vi "vPage_9234x1_CHx4_demo.vi"() -> ()   [LabVIEW 2022 SP3]
uses:
  <vilib>/Utility/sysdir.llb/System Directory Type.ctl
  <vilib>/express/express analysis/Spectral/Block/exnSpectralBlock spectral measurements peak poly.vi
  <vilib>/express/express analysis/Spectral/Block/exnSpectralBlock spectral measurements peak DDT.vi
  <vilib>/express/express analysis/Spectral/XNode/ExpressSpectralMeasurementsBlockNode.xnode
panel:
  out "SPC ALARM":bool
  in  "MTIG":bool
  out "C1":i32
  in  "Show_FFT":bool
  in  "Show":bool
  in  "¸ê®Æ§¨\nµù°O>":string
  in  "Filter(Hz)\nLow-Cut":dbl=10.0
  out "DAQ Stoped":bool
  in  "Sample \nto Read":i32=25600
  in  "Sample\nRate":dbl=25600.0
  in  "Enable Saving":bool
  in  "Stop":bool
  out "C1-Save":bool
  out "C1-Trigger":bool
  out "C1-All":dynamicdata(graph)
  out "C1-0":dynamicdata(graph)
  out "C1-1":dynamicdata(graph)
  out "C1-2":dynamicdata(graph)
  out "C1-3":dynamicdata(graph)
  out "RMS":T1(graph)
  out "P2P":T1(graph) caption="Peak2Peak"
  out "疊層訊號":dbl[][](graph)
  # "使用前請先確認 \nDAQ 擷取卡設定"
  # "本頁畫面顯示為 觸發後訊號"
  # "FFT Filter by useing High-pass with Lower Cut-Off (Hz)"
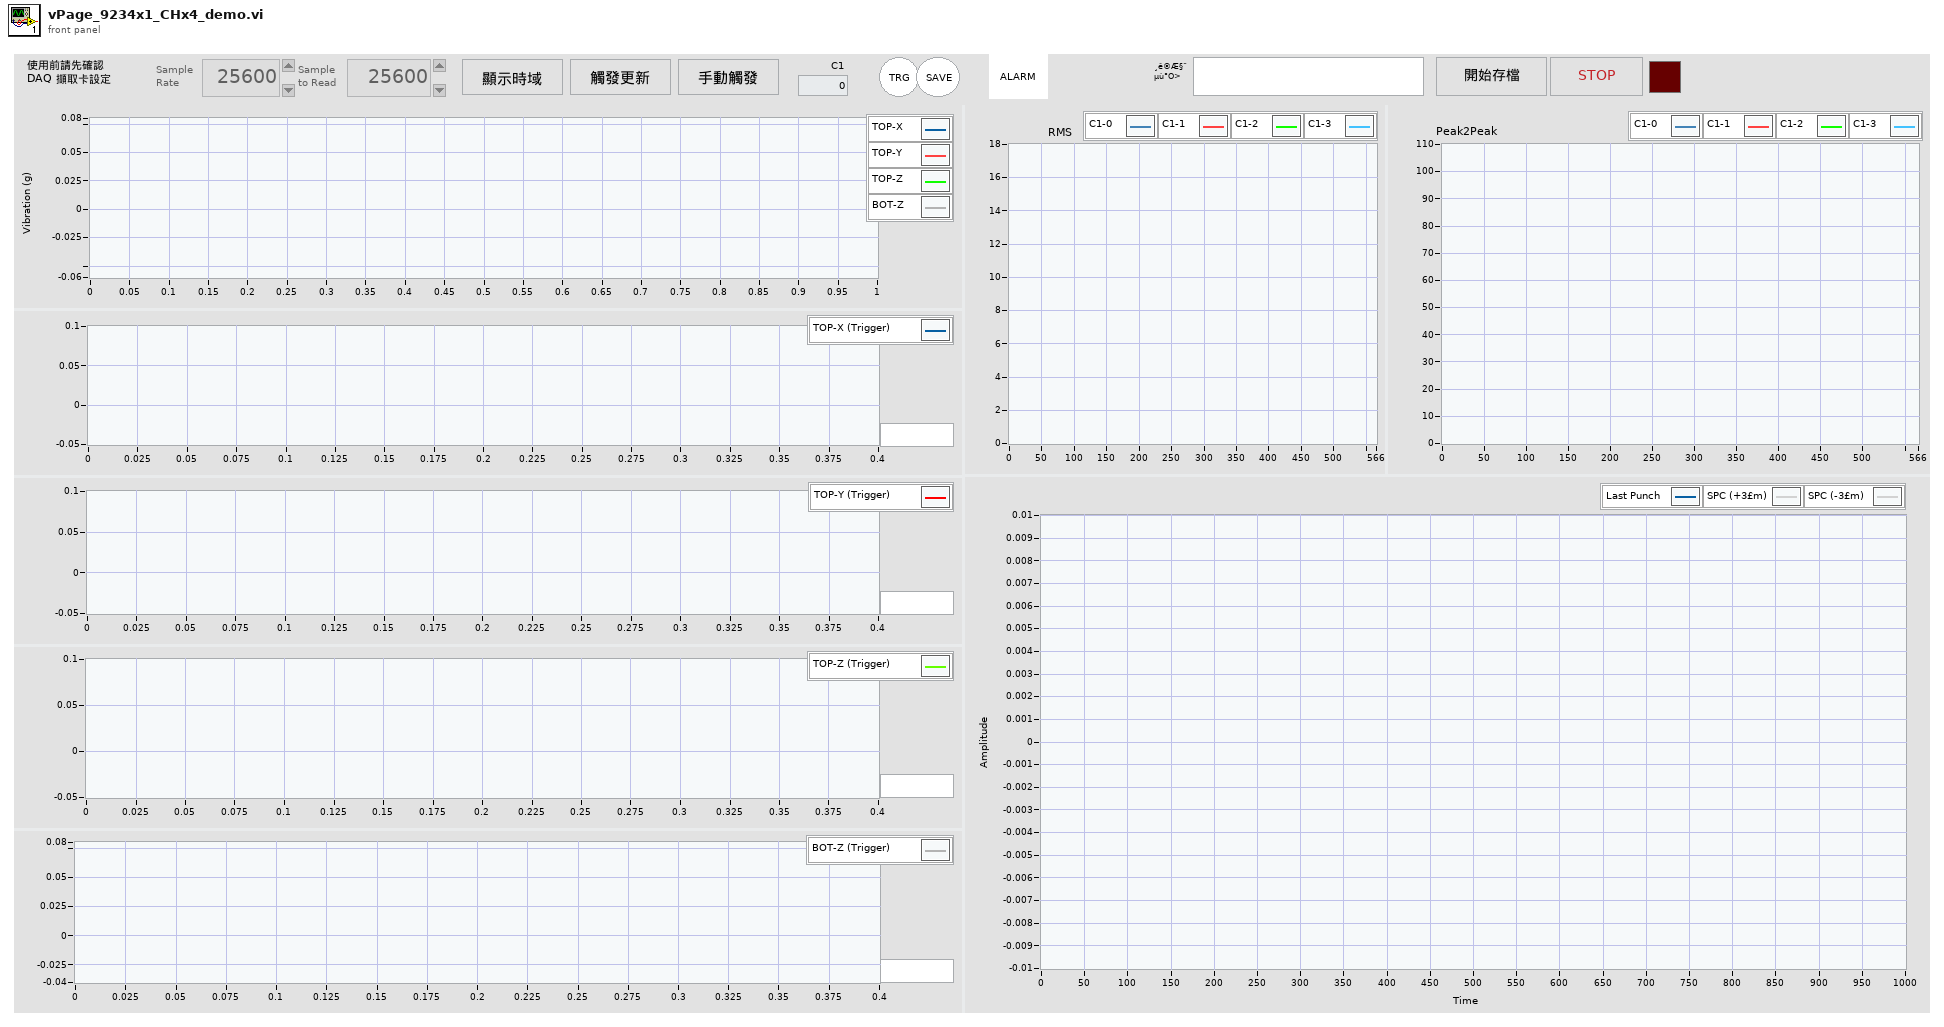
[diagram p1: front panel]
types:
  T1 = cluster{"Array[0]":dbl, "Array[1]":dbl, "Array[2]":dbl, "Array[3]":dbl}
  T2 = enum8{"Enabled", "Disabled", "Disabled and Grayed Out"}
  T3 = typedef "System Directory Type.ctl" = i32
  T4 = cluster{"task out":refnum<k21>, "data":dynamicdata}
  T5 = cluster{"averaging mode":u16, "weighting mode":u16, "number of averages":u32}
  T6 = cluster{"dB On (F)":bool, "unwrap phase (F)":bool, "convert to degree (F)":bool}
  T7 = cluster{"Array[0]":dbl, "Array[1]":dbl, "Array[2]":dbl, "Array[3]":dbl}[]
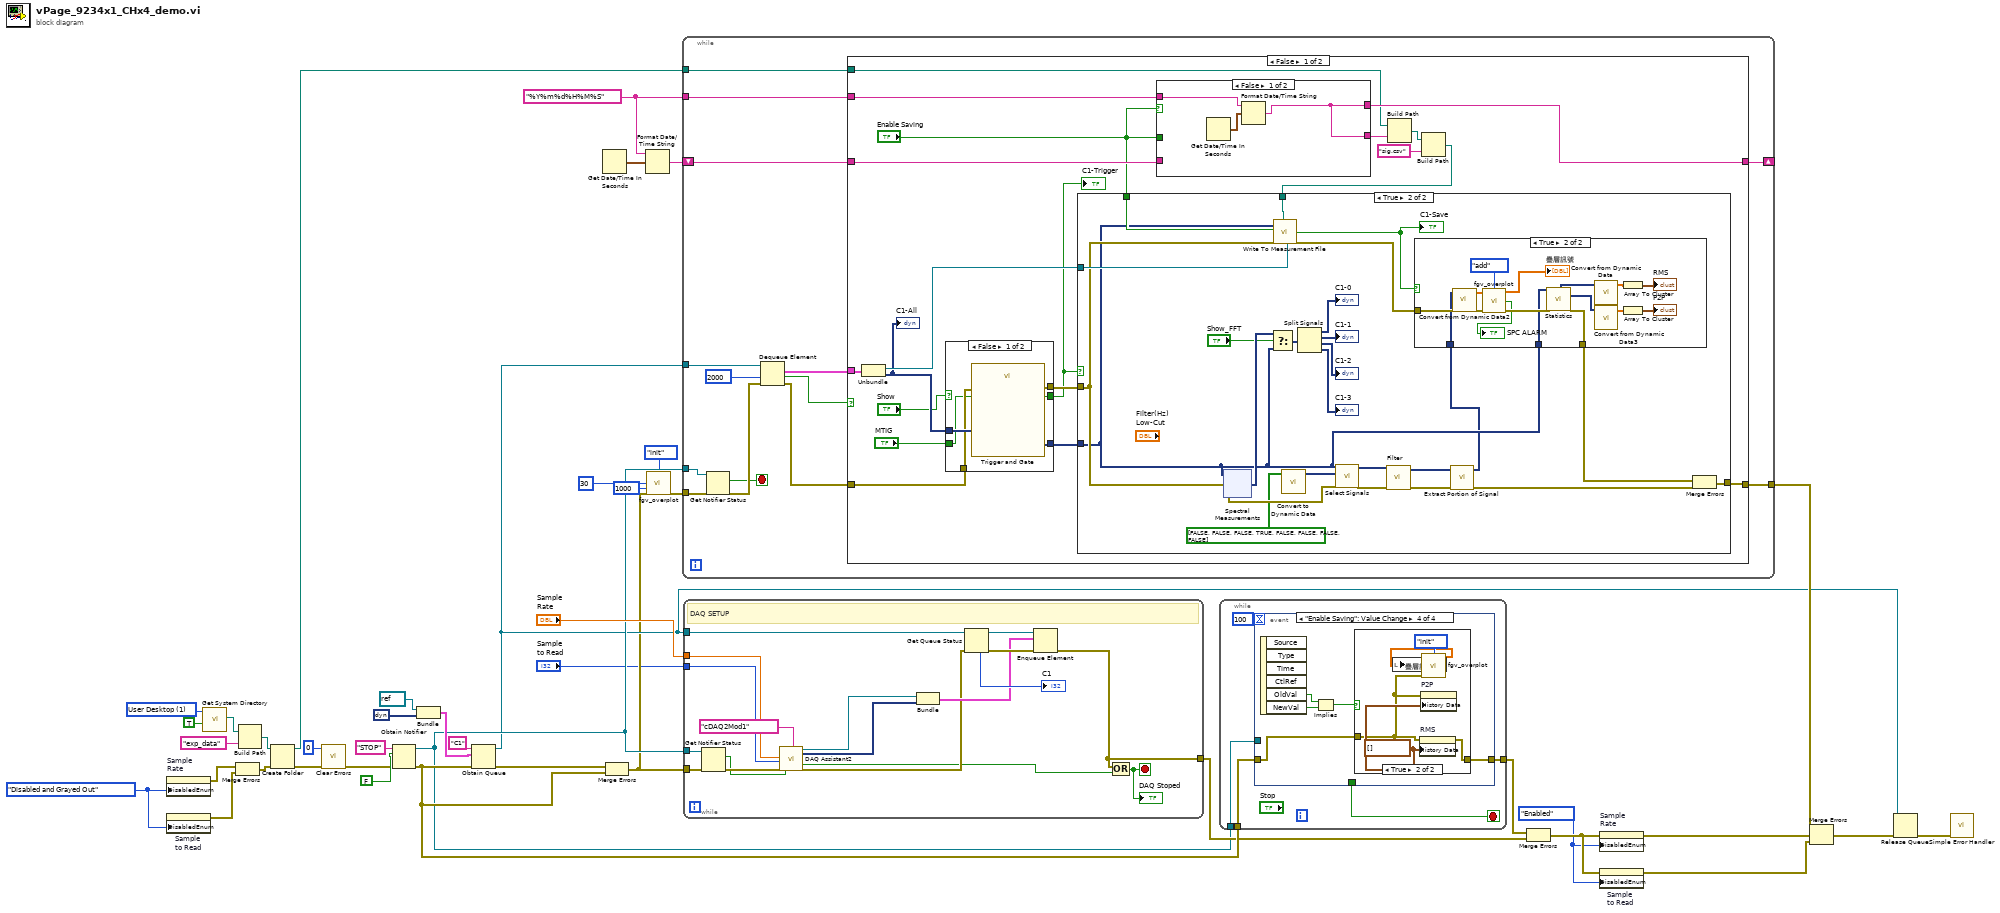
[diagram p0: block diagram]
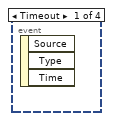
[diagram p2: hidden frame]
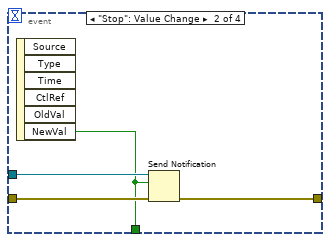
[diagram p3: hidden frame]
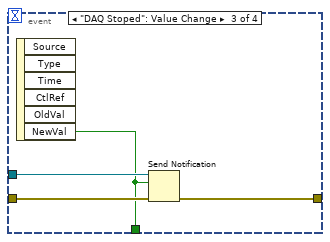
[diagram p4: hidden frame]
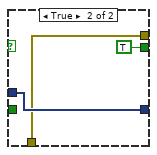
[diagram p8: hidden frame]
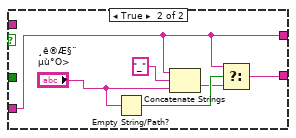
[diagram p9: hidden frame]
diagram:
  w13 = T2."Enabled" ("Disabled")
  w18 = T2."Disabled and Grayed Out" ("Disabled")
  w19 = "%Y%m%d%H%M%S" ("time format string (%c)")
  w29 = T3 1 items=["User Home"=0, "User Desktop"=1, "User Documents"=2, "User Application Data"=3, "User Preferences"=4, "User Temporary"=5, "Public Documents"=6, "Public Application Data"=7, "Public Preferences"=8, "Public Cache"=13, "System Core Libraries"=9, "System Installed Libraries"=10, "Application Files"=11, "Boot Volume Root"=12] ("system directory type")
  n1 = property on="Sample\nRate" class="DigNum (strict)"("DisabledEnum"=w18) -> (error out=w17:errorcluster)  [unwired: 2 in, 1 out]
  n2 = property on="Sample \nto Read" class="DigNum (strict)"("DisabledEnum"=w18) -> (error out=w15:errorcluster)  [unwired: 2 in, 1 out]
  n3 = call <vilib>:"Get System Directory.vi"("create directory if not found? (F)"=TRUE, "system directory type"=w29) -> ("system directory"=w31:path)  [unwired: 9 in]
  n4 = Merge Errors(w17, w15) -> (w16:errorcluster)
  n5 = Build Path(base path=w31, name or relative path="exp_data") -> (appended path=w25:path)
  n6 = Create Folder(path (use dialog)=w25, error in=w16) -> (created path=w24:path, error out=w27:errorcluster)  [unwired: 1 in, 1 out]
  n7 = call <vilib>:"Clear Errors.vi"("error in (no error)"=w27, "specific error code to clear (0: all)"=0) -> ("error out"=w26:errorcluster)  [unwired: 4 in, 1 out]
  n8 = Obtain Notifier(name (unnamed)="STOP", notification data type=FALSE, error in (no error)=w26) -> (notifier out=w20:refnum<notifier>, error out=w23:errorcluster)  [unwired: 1 in, 1 out]
  n9 = Bundle("task out"=refnum<k21> refnum, "data"=dynamicdata []) -> (w35:T4)  [unwired: 1 in]
  n10 = Obtain Queue(name (unnamed)="C1", element data type=w35, error in (no error)=w23) -> (queue out=w7:refnum<queue>, error out=w42:errorcluster)  [unwired: 2 in, 1 out]
  n11 = Get Date/Time In Seconds() -> (seconds since 1Jan1904=w34:timestamp)
  n12 = Merge Errors(w42, w23) -> (w5:errorcluster)
  n13 = Format Date/Time String(time format string (%c)=w19, seconds (now)=w34) -> (date/time string=w33:string)  [unwired: 1 in]
  n14 = call "fgv_overplot.vi"("function (default: show)"=enum16{"init", "add"}."init", "num for avg"=u32 30, "total samples"=u32 1000, "error in"=w5) -> ("error out"=w4:errorcluster)  [unwired: 9 in, 2 out]
  n15 = while {
    tunnel: w4 -> [w56]
    tunnel: w20 -> [w54]
    tunnel: w7 -> [w53]
    shift-right: [w43] -> _
    shift-left: w33 -> [w47]
    tunnel: w24 -> [w48]
    tunnel: [w44] -> w8
    tunnel: w19 -> [w46]
    stop <- w51 stop-if-true
    n16 = Get Notifier Status(notifier=w54, error in (no error)=w56) -> (current notification=w51:bool, error out=w55:errorcluster)  [unwired: 3 out]
    n17 = Dequeue Element(queue=w53, timeout in ms (-1)=2000, error in (no error)=w55) -> (element=w49:T4, timed out?=w50:bool, error out=w45:errorcluster)  [unwired: 1 out]
    n18 = case shown="False" w50 {
      tunnel: w49 -> [w75 _]
      tunnel: w45 -> [w62 w146]
      tunnel: w47 -> [w73 w147]
      tunnel: [w72 w147] -> w43
      tunnel: w48 -> [w71 _]
      tunnel: [w67 w146] -> w44
      tunnel: w46 -> [w65 _]
      frame False {
        n19 = Unbundle(w75) -> ("task out"=w74:refnum<k21>, "data"=w64:dynamicdata)
        "C1-All" <- w64
        n20 = case shown="False" "Show" {
          tunnel: w64 -> [w133 w136]
          tunnel: [w132 w136] -> w63
          tunnel: w62 -> [w131 w135]
          tunnel: [w130 w135] -> w61
          tunnel: [w129 TRUE ("Data Available")] -> w57
          tunnel: "MTIG" -> [w128 _]
          frame False {
            n21 = call "Trigger and Gate"("Manual Trigger"=w128, "error in (no error)"=w131, "Signals"=w133) -> ("error out"=w130:errorcluster, "Triggered Signals"=w132:dynamicdata, "Data Available"=w129:bool)  [unwired: 5 in, 1 out]
          }
          frame True {
          }
        }
        "C1-Trigger" <- w57
        n22 = case shown="False" "Enable Saving" {
          tunnel: [w137 w141] -> w72
          tunnel: "Enable Saving" -> [_ _]
          tunnel: w73 -> [_ w141]
          tunnel: [w137 w143] -> w66
          tunnel: w65 -> [w138 _]
          frame False {
            n23 = Get Date/Time In Seconds() -> (seconds since 1Jan1904=w139:timestamp)
            n24 = Format Date/Time String(time format string (%c)=w138, seconds (now)=w139) -> (date/time string=w137:string)  [unwired: 1 in]
          }
          frame True {
            n25 = Empty String/Path?(string/path="¸ê®Æ§¨\nµù°O>") -> (empty?=w145:bool)
            n26 = Concatenate Strings(w141, "_" ("string"), "¸ê®Æ§¨\nµù°O>") -> (w144:string)
            n27 = Select(t=w141, s=w145, f=w144) -> (s? t:f=w143:string)
          }
        }
        n28 = Build Path(base path=w71, name or relative path=w66) -> (appended path=w70:path)
        n29 = Build Path(base path=w70, name or relative path="sig.csv") -> (appended path=w68:path)
        n30 = case shown="True" w57 {
          tunnel: w74 -> [_ w101]
          tunnel: w68 -> [_ w100]
          tunnel: [w76 w99] -> w67
          tunnel: w63 -> [_ w83]
          tunnel: w61 -> [w76 w84]
          tunnel: "Enable Saving" -> [_ w91]
          frame False {
          }
          frame True {
            n31 = xnode ("Spectral Measurements")("Signals"=w83, "error in (no error)"=w84) -> ("FFT - (Peak)"=w98:dynamicdata, "error out"=w94:errorcluster)  [unwired: 1 out]
            n32 = Select(t=w98, s="Show_FFT", f=w83) -> (s? t:f=w97:dynamicdata)
            n33 = call "Write To Measurement File"("Signals"=w83, "Enable"=w91, "error in (no error)"=w84, "Filename"=w100, "DAQmx Task"=w101) -> ("Saving Data"=w85:bool, "error out"=w86:errorcluster)  [unwired: 12 in, 1 out]
            "C1-Save" <- w85
            n34 = call "Convert to Dynamic Data"("Array"=bool[] [FALSE, FALSE, FALSE, TRUE, FALSE, FALSE, FALSE, FALSE] ("SW \n(C1)")) -> ("Dynamic Data Type"=w92:dynamicdata)  [unwired: 3 in]
            n35 = Split Signals(w97) -> (→"C1-0":dynamicdata, →"C1-1":dynamicdata, →"C1-2":dynamicdata, →"C1-3":dynamicdata)  [unwired: 4 in]
            n36 = call "Select Signals"("error in (no error)"=w94, "Selector Input"=w92, "Signals"=w83) -> ("error out"=w77:errorcluster, "Signal Out"=w81:dynamicdata)  [unwired: 7 in]
            n37 = call "Filter"("error in (no error)"=w77, "Signal"=w81) -> ("error out"=w82:errorcluster, "Filtered Signal"=w80:dynamicdata)  [unwired: 8 in]
            n38 = call "Extract Portion of Signal"("error in (no error)"=w82, "Signals"=w80) -> ("error out"=w78:errorcluster, "Section"=w79:dynamicdata)  [unwired: 8 in]
            n39 = case shown="True" w85 {
              tunnel: [w102 w114] -> w95
              tunnel: w86 -> [w102 w107]
              tunnel: w79 -> [_ w105]
              tunnel: w83 -> [_ w104]
              frame False {
              }
              frame True {
                n40 = call "Convert from Dynamic Data2"("Dynamic Data Type"=w105) -> ("Array"=w112:dbl[])  [unwired: 3 in]
                n41 = call "fgv_overplot.vi"("Data in"=w112, "function (default: show)"=enum16{"init", "add", "show"}."add", "error in"=w107) -> ("Plot"=→"疊層訊號":dbl[][], "SPC ALARM"=→"SPC ALARM":bool, "error out"=w106:errorcluster)  [unwired: 10 in]
                n42 = call "Statistics"("Signals"=w104, "error in (no error)"=w106) -> ("RMS"=w117:dynamicdata, "Range"=w110:dynamicdata, "error out"=w114:errorcluster)  [unwired: 23 in]
                n43 = call "Convert from Dynamic Data"("Dynamic Data Type"=w117) -> ("Array"=w116:dbl[])  [unwired: 3 in]
                n44 = call "Convert from Dynamic Data3"("Dynamic Data Type"=w110) -> ("Array"=w111:dbl[])  [unwired: 3 in]
                n45 = Array To Cluster(array=w116) -> (cluster=→"RMS":T1)
                n46 = Array To Cluster(array=w111) -> (cluster=→"P2P":T1)
              }
            }
            n47 = Merge Errors(w95, w78) -> (w99:errorcluster)
          }
        }
      }
      frame True {
      }
    }
  }
  n48 = while {
    tunnel: [w164] -> w21
    tunnel: w7 -> [w161]
    tunnel: w5 -> [w160]
    tunnel: w20 -> [w159]
    tunnel: "Sample \nto Read" -> [w153]
    tunnel: "Sample\nRate" -> [w154]
    stop <- w162 stop-if-true
    # "DAQ SETUP"
    n49 = Get Notifier Status(notifier=w159, error in (no error)=w160) -> (current notification=w152:bool, error out=w156:errorcluster)  [unwired: 3 out]
    n50 = call "DAQ Assistant2"("rate"=w154, "number of samples"=w153, "error in"=w156, "stop (F)"=w152, "device name"=tag "cDAQ2Mod1") -> ("task out"=w150:refnum<k21>, "data"=w149:dynamicdata, "stopped"=w151:bool, "error out"=w155:errorcluster)  [unwired: 11 in]
    n51 = Bundle("task out"=w150, "data"=w149) -> (w157:T4)  [unwired: 1 in]
    n52 = Get Queue Status(queue=w161, error in (no error)=w155) -> (queue out=w158:refnum<queue>, error out=w165:errorcluster, # elements in queue=→"C1":i32)  [unwired: 1 in, 5 out]
    n53 = Enqueue Element(queue=w158, element=w157, error in (no error)=w165) -> (error out=w164:errorcluster)  [unwired: 1 in, 2 out]
    n54 = Compound Arithmetic op=OR(w164, w151) -> (w162:bool)
    "DAQ Stoped" <- w162
  }
  n55 = while {
    tunnel: w23 -> [w170]
    tunnel: [w169] -> w22
    tunnel: w20 -> [w168]
    stop <- w167 stop-if-true
    n56 = event shown="[3] \"Enable Saving\": Value Change" {
      selector: _ -> [_ _ _ _]
      dyn-events: _ -> [_ _ _ _]
      timeout: 100 -> [_ _ _ _]
      tunnel: w170 -> [_ w174 w178 w181]
      tunnel: [_ w173 w177 w180] -> w169
      tunnel: w168 -> [_ w172 w176 _]
      tunnel: [_ w171 w175 _] -> w167
      event Timeout {
        n57 = event-data() -> ()  [unwired: 1 in, 3 out]
      }
      event "Stop": Value Change {
        n58 = event-data() -> ("NewVal"=w171:bool)  [unwired: 1 in, 5 out]
        n59 = Send Notification(notification=w171, notifier=w172, error in (no error)=w174) -> (error out=w173:errorcluster)  [unwired: 1 out]
      }
      event "DAQ Stoped": Value Change {
        n60 = event-data() -> ("NewVal"=w175:bool)  [unwired: 1 in, 5 out]
        n61 = Send Notification(notification=w175, notifier=w176, error in (no error)=w178) -> (error out=w177:errorcluster)  [unwired: 1 out]
      }
      event "Enable Saving": Value Change {
        n62 = event-data() -> ("OldVal"=w182:bool, "NewVal"=w183:bool)  [unwired: 1 in, 4 out]
        n63 = Implies(1:w183, 2:w182) -> (0:w179:bool)
        n64 = case shown="True" w179 {
          tunnel: w181 -> [w184 w186]
          tunnel: [w184 w189] -> w180
          frame False {
          }
          frame True {
            w188 = T7 [] ("History Data")
            n65 = property on="RMS" class="WFChart (strict)"(error in=w186, "History Data"=w188) -> (error out=w189:errorcluster)  [unwired: 1 in, 1 out]
            n66 = property on="P2P" class="WFChart (strict)"(error in=w186, "History Data"=w188) -> ()  [unwired: 1 in, 2 out]
            n67 = call "fgv_overplot.vi"("function (default: show)"=enum16{"init", "add"}."init", "error in"=w186) -> ("Plot"=w185:dbl[][])  [unwired: 11 in, 2 out]
            n68 = local write "疊層訊號"(w185) -> ()
          }
        }
      }
    }
  }
  n69 = Merge Errors(w22, w21) -> (w14:errorcluster)
  n70 = property on="Sample\nRate" class="DigNum (strict)"(error in=w14, "DisabledEnum"=w13) -> (error out=w12:errorcluster)  [unwired: 1 in, 1 out]
  n71 = property on="Sample \nto Read" class="DigNum (strict)"(error in=w14, "DisabledEnum"=w13) -> (error out=w11:errorcluster)  [unwired: 1 in, 1 out]
  n72 = Merge Errors(w8, w12, w11) -> (w9:errorcluster)
  n73 = Release Queue(queue=w7, error in (no error)=w9) -> (error out=w10:errorcluster)  [unwired: 1 in, 2 out]
  n74 = call <vilib>:"Simple Error Handler.vi"("error in (no error)"=w10) -> ()  [unwired: 4 in, 5 out]
